vi "Read datatype.vi"(8 "error in (no error)":errorcluster, 11 "PointerDatatype in":refnum<class "PointerDatatype.lvclass">) -> (0 "error out":errorcluster, 2 "datatype":string, 3 "PointerDatatype out":refnum<class "PointerDatatype.lvclass">)   [LabVIEW 2014, in "PointerDatatype.lvclass"]
uses:
  PointerDatatype.lvclass
  PointerDatatype.lvclass/PointerDatatype.ctl
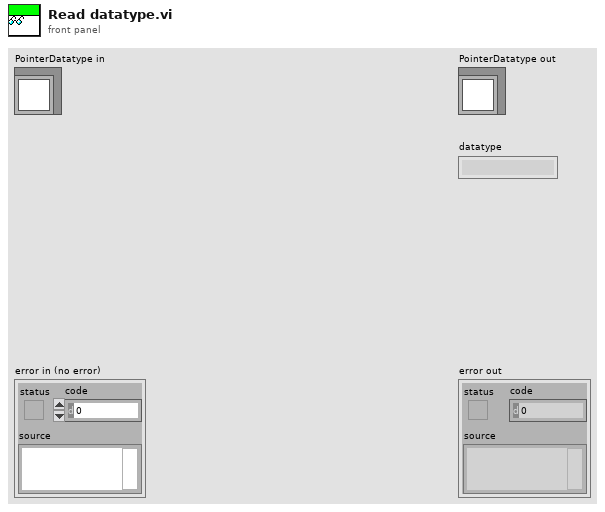
[diagram p1: front panel]
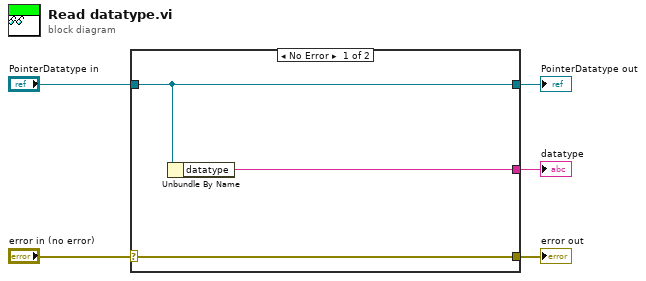
[diagram p0: block diagram]
diagram:
  n1 = case shown="No Error" "error in (no error)" {
    selector: "error in (no error)" -> [w8 w9]
    tunnel: [w8 w9] -> w4
    tunnel: [w7 w10] -> w2
    tunnel: "PointerDatatype in" -> [w7 w10]
    tunnel: [w6 _] -> w1
    frame No Error {
      n2 = Unbundle By Name(w7) -> ("datatype"=w6:string)
    }
    frame Error {
    }
  }
  "error out" <- w4
  "PointerDatatype out" <- w2
  "datatype" <- w1
